vi "markMFCsRequired.vi"(9 "suggestedCombo":T1[](array[typedef]), 11 "MFCsIn":T1[](array[typedef])) -> (3 "MFCsOut":T1[](array[typedef]))   [LabVIEW 2016]
uses:
  MFCdescription.ctl
  MFCcapability.ctl
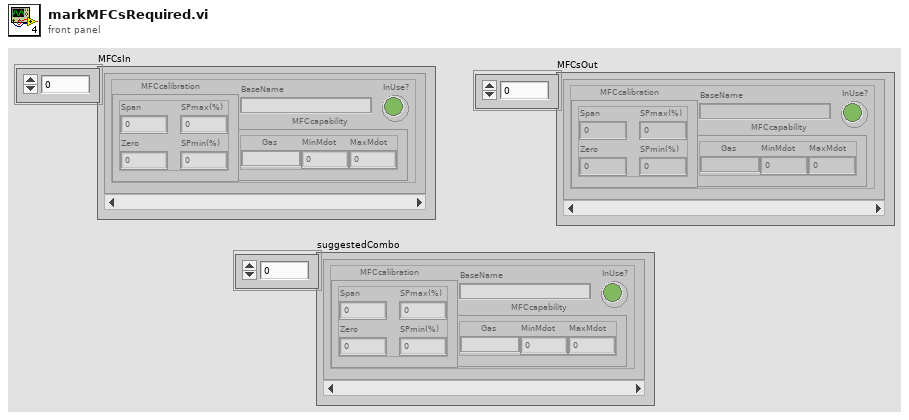
[diagram p1: front panel]
types:
  T1 = typedef "MFCdescription.ctl" = cluster{"BaseName":string, "MFCcalibration":cluster{"Span":dbl, "Zero":dbl, "SPmin(%)":dbl, "SPmax(%)":dbl}, "MFCcapability":T2, "InUse?":bool}
  T2 = typedef "MFCcapability.ctl" = cluster{"Gas":string, "MinMdot":dbl, "MaxMdot":dbl}
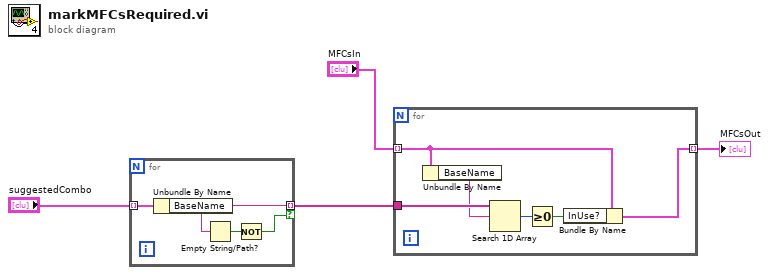
[diagram p0: block diagram]
diagram:
  n1 = for {
    tunnel: "suggestedCombo" -> [w8] mode=indexing
    tunnel: [w7] -> w1 mode=indexing if=w5
    n2 = Unbundle By Name(w8) -> ("BaseName"=w7:string)
    n3 = Empty String/Path?(string/path=w7) -> (empty?=w6:bool)
    n4 = Not(x=w6) -> (.not. x?=w5:bool)
  }
  n5 = for {
    tunnel: [w10] -> w2 mode=indexing
    tunnel: "MFCsIn" -> [w11] mode=indexing
    tunnel: w1 -> [w14]
    n6 = Unbundle By Name(w11) -> ("BaseName"=w13:string)
    n7 = Search 1D Array(1D array=w14, element=w13) -> (index of element=w12:i32)  [unwired: 1 in]
    n8 = Greater Or Equal To 0?(x=w12) -> (x >= 0?=w9:bool)
    n9 = Bundle By Name(cluster=w11, "InUse?"=w9) -> (w10:T1)
  }
  "MFCsOut" <- w2
